vi "settings.vi"(8 "Error In":errorcluster) -> (0 "Error Out":errorcluster)   [LabVIEW 2012]
uses:
  Scanning Setting.vi
panel:
  in  "1000Hz":bool
  in  "30fps":bool
  in  "100fps":bool
  in  "Single line Scan":bool
  in  "Default":bool
  in  "S Angle Correction (ratio)":dbl(knob)=-0.29473162999791414 scale=-0.5..0.5
  in  "Z-offset":dbl(slide)=-1.748502994011976 scale=-4.0..4.0
  in  "Cancel Button":bool
  in  "OK Button":bool
  in  "S-offset":dbl(slide)=-1.8947368421052633 scale=-4.0..4.0
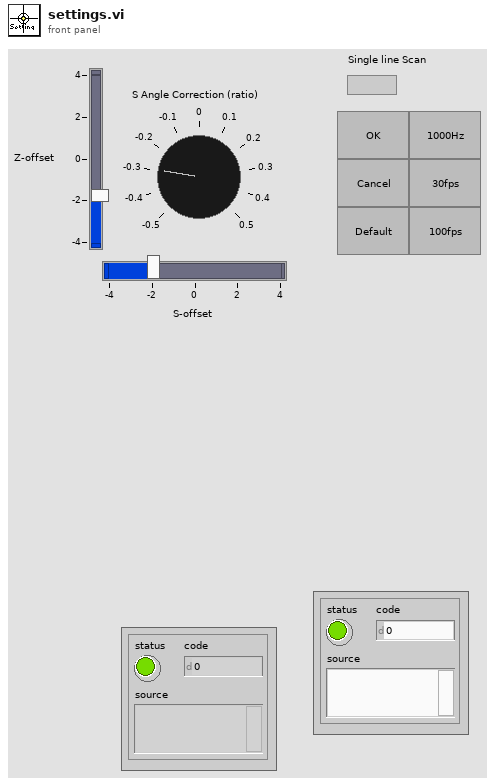
[diagram p1: front panel]
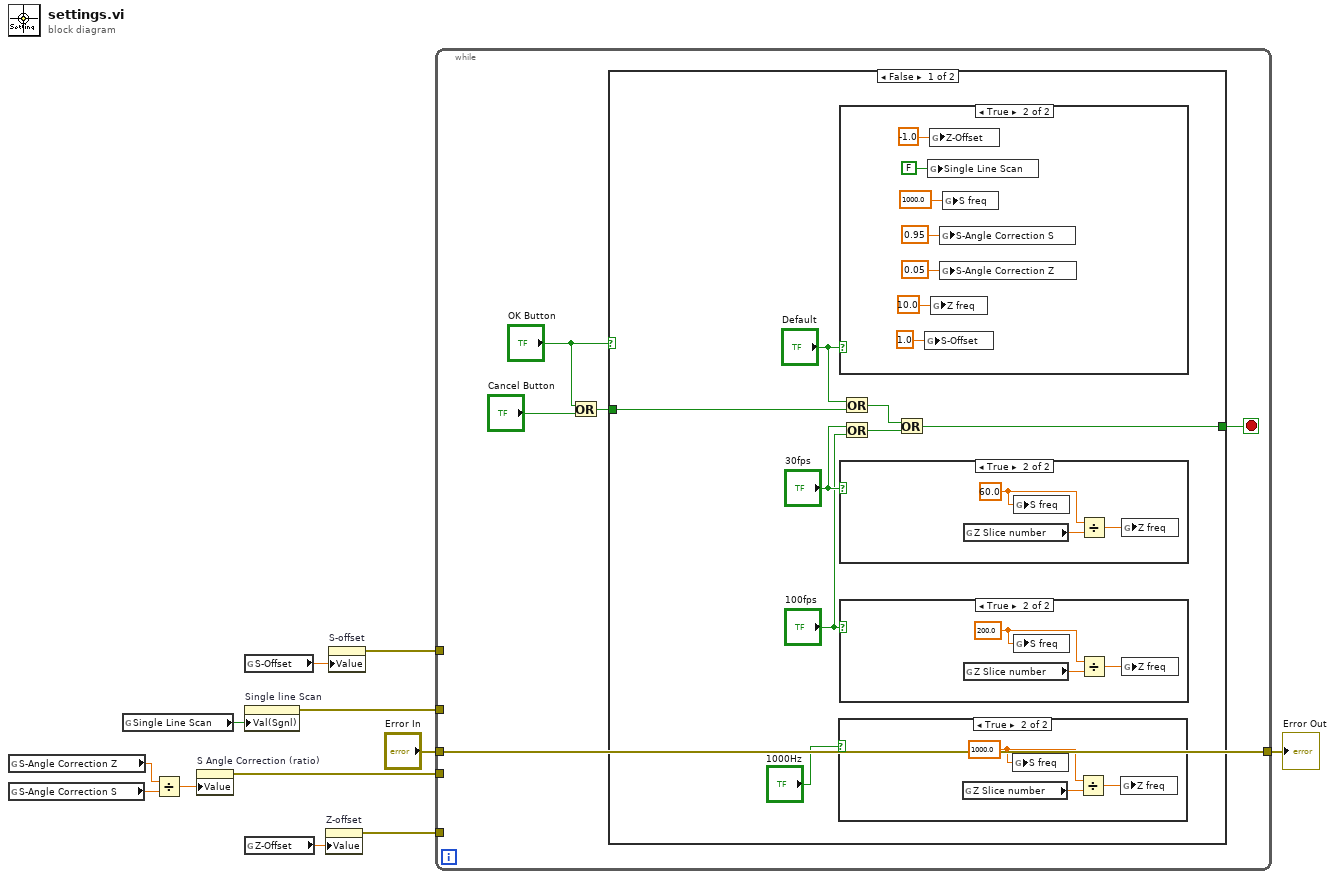
[diagram p0: block diagram]
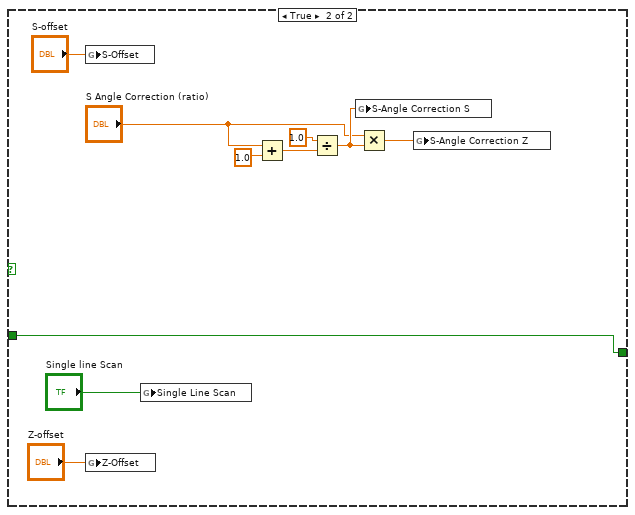
[diagram p6: hidden frame]
diagram:
  n1 = global read "Scanning Setting.vi" "S-Angle Correction Z"() -> (w6:dbl)
  n2 = global read "Scanning Setting.vi" "S-Angle Correction S"() -> (w5:dbl)
  n3 = global read "Scanning Setting.vi" "Single Line Scan"() -> (w2:bool)
  n4 = Divide(x=w6, y=w5) -> (x/y=w4:dbl)
  n5 = property on="S Angle Correction (ratio)" class="Knob (strict)"("Value"=w4) -> (error out=w3:errorcluster)  [unwired: 2 in, 1 out]
  n6 = global read "Scanning Setting.vi" "S-Offset"() -> (w12:dbl)
  n7 = property on="Single line Scan" class="Bool (strict)"("Val(Sgnl)"=w2) -> (error out=w1:errorcluster)  [unwired: 2 in, 1 out]
  n8 = global read "Scanning Setting.vi" "Z-Offset"() -> (w10:dbl)
  n9 = property on="Z-offset" class="Slide (strict)"("Value"=w10) -> (error out=w9:errorcluster)  [unwired: 2 in, 1 out]
  n10 = property on="S-offset" class="Slide (strict)"("Value"=w12) -> (error out=w11:errorcluster)  [unwired: 2 in, 1 out]
  n11 = while {
    tunnel: w11 -> [_]
    tunnel: w9 -> [_]
    tunnel: "Error In" -> [w13]
    tunnel: [w13] -> w7
    tunnel: w3 -> [_]
    tunnel: w1 -> [_]
    stop <- w14 stop-if-true
    n12 = Or(x="OK Button", y="Cancel Button") -> (x .or. y?=w15:bool)
    n13 = case shown="False" "OK Button" {
      tunnel: w15 -> [w24 w50]
      tunnel: [w19 w50] -> w14
      frame False {
        n14 = case shown="True" "1000Hz" {
          frame False {
          }
          frame True {
            w28 = 1000.0 ("S freq")
            n15 = global read "Scanning Setting.vi" "Z Slice number"() -> (w27:dbl)
            n16 = global write "Scanning Setting.vi" "S freq"(w28) -> ()
            n17 = Divide(x=w28, y=w27) -> (x/y=w26:dbl)
            n18 = global write "Scanning Setting.vi" "Z freq"(w26) -> ()
          }
        }
        n19 = case shown="True" "Default" {
          frame False {
          }
          frame True {
            n20 = global write "Scanning Setting.vi" "S-Offset"(1.0 ("S-Offset")) -> ()
            n21 = global write "Scanning Setting.vi" "Single Line Scan"(FALSE ("Single Line Scan")) -> ()
            n22 = global write "Scanning Setting.vi" "Z-Offset"(-1.0 ("Z-Offset")) -> ()
            n23 = global write "Scanning Setting.vi" "Z freq"(10.0 ("Z freq")) -> ()
            n24 = global write "Scanning Setting.vi" "S-Angle Correction S"(0.95 ("S-Angle Correction S")) -> ()
            n25 = global write "Scanning Setting.vi" "S-Angle Correction Z"(0.05 ("S-Angle Correction Z")) -> ()
            n26 = global write "Scanning Setting.vi" "S freq"(1000.0 ("S freq")) -> ()
          }
        }
        n27 = case shown="True" "30fps" {
          frame False {
          }
          frame True {
            w34 = 60.0 ("S freq")
            n28 = global read "Scanning Setting.vi" "Z Slice number"() -> (w33:dbl)
            n29 = global write "Scanning Setting.vi" "S freq"(w34) -> ()
            n30 = Divide(x=w34, y=w33) -> (x/y=w32:dbl)
            n31 = global write "Scanning Setting.vi" "Z freq"(w32) -> ()
          }
        }
        n32 = case shown="True" "100fps" {
          frame False {
          }
          frame True {
            w31 = 200.0 ("S freq")
            n33 = global read "Scanning Setting.vi" "Z Slice number"() -> (w30:dbl)
            n34 = global write "Scanning Setting.vi" "S freq"(w31) -> ()
            n35 = Divide(x=w31, y=w30) -> (x/y=w29:dbl)
            n36 = global write "Scanning Setting.vi" "Z freq"(w29) -> ()
          }
        }
        n37 = Or(x="Default", y=w24) -> (x .or. y?=w20:bool)
        n38 = Or(x="30fps", y="100fps") -> (x .or. y?=w21:bool)
        n39 = Or(x=w20, y=w21) -> (x .or. y?=w19:bool)
      }
      frame True {
        n40 = global write "Scanning Setting.vi" "S-Offset"("S-offset") -> ()
        n41 = global write "Scanning Setting.vi" "Z-Offset"("Z-offset") -> ()
        n42 = global write "Scanning Setting.vi" "Single Line Scan"("Single line Scan") -> ()
        n43 = Add(x="S Angle Correction (ratio)", y=1.0) -> (x+y=w47:dbl)
        n44 = Divide(x=1.0, y=w47) -> (x/y=w45:dbl)
        n45 = global write "Scanning Setting.vi" "S-Angle Correction S"(w45) -> ()
        n46 = Multiply(x="S Angle Correction (ratio)", y=w45) -> (x*y=w43:dbl)
        n47 = global write "Scanning Setting.vi" "S-Angle Correction Z"(w43) -> ()
      }
    }
  }
  "Error Out" <- w7
